vi "禁用控件.vi"(6 "控件组":refnum<vi>[](array[refnum]), 7 "禁用？(F)":bool, 8 "错误输入（无错误）":errorcluster) -> (0 "错误输出":errorcluster)   [LabVIEW 2021]
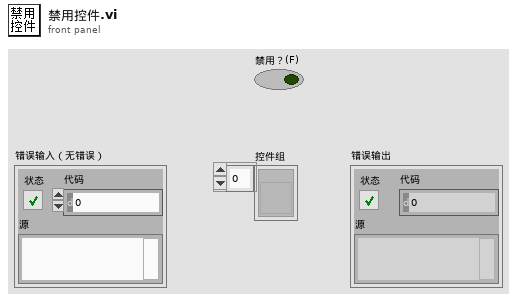
[diagram p1: front panel]
types:
  T1 = enum8{"Enabled", "Disabled", "Disabled and Grayed Out"}
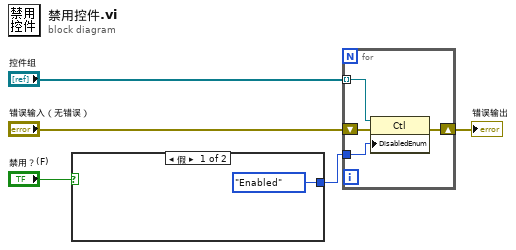
[diagram p0: block diagram]
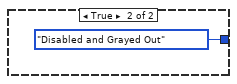
[diagram p2: hidden frame]
diagram:
  n1 = case shown="假" "禁用？(F)" {
    tunnel: [T1."Enabled" ("禁用") T1."Disabled and Grayed Out" ("禁用")] -> w4
    frame False {
    }
    frame True {
    }
  }
  n2 = for {
    tunnel: w4 -> [w10]
    shift-right: [w8] -> w2
    shift-left: "错误输入（无错误）" -> [w11]
    tunnel: "控件组" -> [w9] mode=indexing
    n3 = property class="Ctl"(reference=w9, error in=w11, "DisabledEnum"=w10) -> (error out=w8:errorcluster)  [unwired: 1 out]
  }
  "错误输出" <- w2
